vi "Read Header and Spreadsheet File.vi"(0 "DirIn":path=path "C:/ER2005/Data", 1 "NameIn":string="Test001.txt", 3 "Headers Only":bool, 4 "# Hdr Lines":i32=23 min=0, 5 "Error In":errorcluster, 6 "File Read Mode":enum16{"Never", "List", "Ask"}(ring)=enum."Ask", 8 "Delimiter (Tab)":string="\t", 10 "Format (%.4f)":string="%.4f", 11 "ErrMsgOff":bool, 13 "Transpose":bool) -> (12 "Table Out":string[][](array[string]), 14 "Filepath Out":path, 15 "File Text Out":string, 16 "Header Lines":string[](array[string]), 17 "Last 1D":sgl[](array[numeric]) format="%.2f", 18 "2D Data":sgl[][](array[numeric]) format="%.2f", 19 "Error Out":errorcluster)   [LabVIEW 2013]
panel:
  # "Err 1 - Invalid input parameter\nErr 4 - End-of-file\nErr 7 - Open error, file does not exist\nErr 43 - Cancel error"
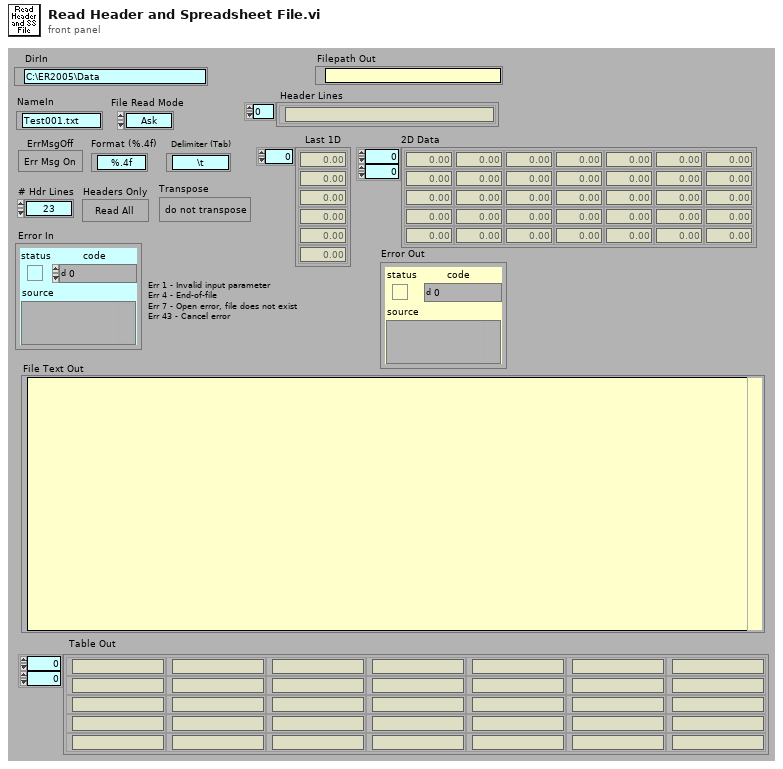
[diagram p1: front panel]
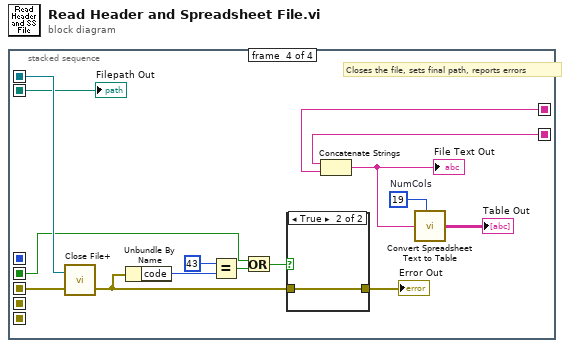
[diagram p0: block diagram]
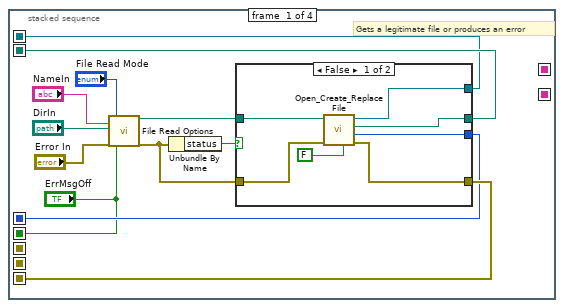
[diagram p2: hidden frame]
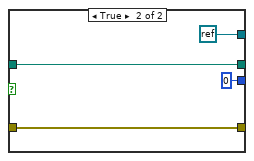
[diagram p3: hidden frame]
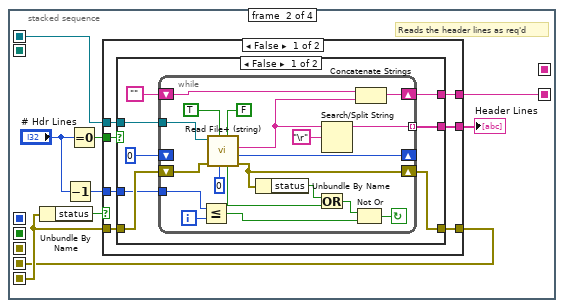
[diagram p4: hidden frame]
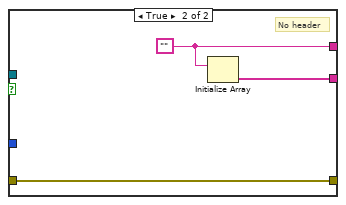
[diagram p5: hidden frame]
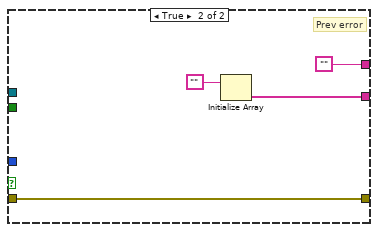
[diagram p6: hidden frame]
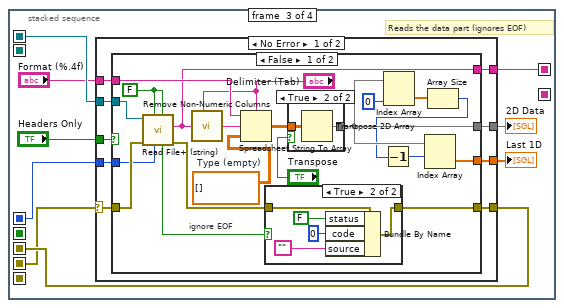
[diagram p7: hidden frame]
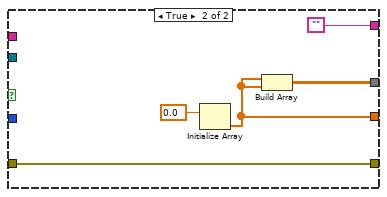
[diagram p10: hidden frame]
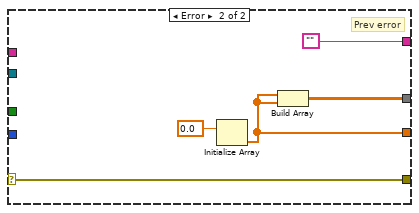
[diagram p11: hidden frame]
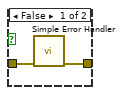
[diagram p12: hidden frame]
diagram:
  n1 = stacked-sequence {
    seq-local: [w5 _ _ _] -> [_ w31 _ _]
    seq-local: [w3 _ _ _] -> [_ w29 w81 w145]
    seq-local: [w4 _ _ _] -> [_ _ _ w144]
    seq-local: [_ w27 _ _] -> [_ _ w74 _]
    seq-local: [_ _ w82 _] -> [_ _ _ w143]
    seq-local: [w2 _ _ _] -> [_ _ w79 _]
    seq-local: ["ErrMsgOff" _ _ _] -> [_ _ _ w137]
    seq-local: [_ w24 _ _] -> [_ _ _ w135]
    seq-local: [_ _ w75 _] -> [_ _ _ w134]
    frame #0 {
      # "Gets a legitimate file or produces an error"
      n2 = call "File Read Options.vi"("NameIn"="NameIn", "DirIn"="DirIn", "ErrorIn (no error)"="Error In", "File Read Mode"="File Read Mode", "ErrMsgOff"="ErrMsgOff") -> ("PathOut"=w6:path, "ErrorOut"=w7:errorcluster)  [unwired: 7 in, 6 out]
      n3 = Unbundle By Name(w7) -> ("status"=w8:bool)
      n4 = case shown="False" w8 {
        tunnel: w6 -> [w19 w21]
        tunnel: [w16 w23] -> w5
        tunnel: w7 -> [w17 w23]
        tunnel: [w15 refnum<k0> refnum] -> w3
        tunnel: [w14 w21] -> w4
        tunnel: [w13 0 ("file size (bytes)")] -> w2
        frame False {
          n5 = call <vilib>:"Open_Create_Replace File.vi"("advisory dialog? (display:T)"=FALSE, "error in (no error)"=w17, "file path"=w19) -> ("error out"=w16:errorcluster, "file size (bytes)"=w13:i32, "new file path"=w14:path, "refnum"=w15:refnum<file>)  [unwired: 5 in]
        }
        frame True {
        }
      }
    }
    frame #1 {
      # "Reads the header lines as req'd"
      n6 = Unbundle By Name(w31) -> ("status"=w32:bool)
      n7 = Decrement(x="# Hdr Lines") -> (x-1=w25:i32)
      n8 = Equal To 0?(x="# Hdr Lines") -> (x = 0?=w30:bool)
      n9 = case shown="False" w32 {
        tunnel: w31 -> [w38 w71]
        tunnel: w25 -> [w37 _]
        tunnel: w30 -> [w39 _]
        tunnel: w29 -> [w36 _]
        tunnel: [w35 w72] -> w28
        tunnel: [w34 w71] -> w27
        tunnel: [w33 ""] -> w24
        frame False {
          n10 = case shown="False" w39 {
            tunnel: w38 -> [w46 w68]
            tunnel: w37 -> [w42 _]
            tunnel: w36 -> [w47 _]
            tunnel: [w44 w69] -> w35
            tunnel: [w43 w68] -> w34
            tunnel: [w40 w67] -> w33
            frame False {
              n11 = while {
                tunnel: w42 -> [w61]
                tunnel: [w51] -> w44 mode=indexing
                shift-left: 0 ("mark after read (bytes)") -> [_]
                shift-right: [w62] -> _
                shift-left: w46 -> [w63]
                shift-right: [w59] -> w43
                tunnel: w47 -> [w64]
                shift-right: [w50] -> w40
                shift-left: "" -> [w49]
                i -> [w60]
                stop <- w57 continue-if-true
                n12 = Less Or Equal?(x=w61, y=w60) -> (x <= y?=w58:bool)
                n13 = call <vilib>:"Read File+ (string).vi"("convert eol? (no:F)"=FALSE, "count"=0, "line mode (characters:F)"=TRUE, "error in (no error)"=w63, "refnum"=w64) -> ("error out"=w59:errorcluster, "mark after read (bytes)"=w62:i32, "string"=w48:string, "EOF?"=w56:bool)  [unwired: 2 in, 1 out]
                n14 = Unbundle By Name(w59) -> ("status"=w55:bool)
                n15 = Or(x=w55, y=w56) -> (x .or. y?=w54:bool)
                n16 = Search/Split String(string=w48, search string/char (-)="\r") -> (substring before match=w51:string)  [unwired: 1 in, 2 out]
                n17 = Not Or(1:w58, 2:w54) -> (0:w57:bool)
                n18 = Concatenate Strings(w49, w48) -> (w50:string)
              }
            }
            frame True {
              w67 = ""
              # "No header"
              n19 = Initialize Array(w67) -> (w69:string[])  [unwired: 1 in]
            }
          }
        }
        frame True {
          # "Prev error"
          n20 = Initialize Array("") -> (w72:string[])  [unwired: 1 in]
        }
      }
      "Header Lines" <- w28
    }
    frame #2 {
      # "Reads the data part (ignores EOF)"
      n21 = case shown="No Error" w74 {
        selector: w74 -> [w83 w126]
        tunnel: "Headers Only" -> [w91 _]
        tunnel: w81 -> [w90 _]
        tunnel: [w89 w126] -> w82
        tunnel: w79 -> [w88 _]
        tunnel: [w87 w129] -> w78
        tunnel: [w86 w128] -> w77
        tunnel: "Format (%.4f)" -> [w85 _]
        tunnel: [w84 ""] -> w75
        frame No Error {
          n22 = case shown="False" w91 {
            tunnel: w83 -> [w110 w125]
            tunnel: w90 -> [w111 _]
            tunnel: [w104 w125] -> w89
            tunnel: w88 -> [w109 _]
            tunnel: [w101 w122] -> w87
            tunnel: [w105 w123] -> w86
            tunnel: w85 -> [w95 _]
            tunnel: [w94 ""] -> w84
            frame False {
              w108 = sgl[][] []  # Type (empty)
              w96 = FALSE ("line mode (characters:F)")
              # "ignore EOF"
              n23 = call <vilib>:"Read File+ (string).vi"("convert eol? (no:F)"=w96, "count"=w109, "line mode (characters:F)"=w96, "error in (no error)"=w110, "refnum"=w111) -> ("error out"=w103:errorcluster, "string"=w94:string, "EOF?"=w102:bool)  [unwired: 2 in, 2 out]
              n24 = call "Remove Non-Numeric Columns.vi"("Separator (Tab)"="Delimiter (Tab)", "String In"=w94) -> ("String Out"=w93:string)  [unwired: 6 in, 1 out]
              n25 = Spreadsheet String To Array(delimiter (Tab)="Delimiter (Tab)", format string=w95, spreadsheet string=w93, array type (2D Dbl)=w108) -> (array=w107:sgl[][])
              n26 = case shown="True" w102 {
                tunnel: [w112 w116] -> w104
                tunnel: w103 -> [w112 w117]
                frame False {
                }
                frame True {
                  n27 = Bundle By Name(cluster=w117, "status"=FALSE ("Bundle Element"), "code"=0 ("Bundle Element"), "source"="") -> (w116:errorcluster)
                }
              }
              n28 = case shown="True" "Transpose" {
                tunnel: w107 -> [w118 w120]
                tunnel: [w118 w119] -> w101
                frame False {
                }
                frame True {
                  n29 = Transpose 2D Array(2D array=w120) -> (transposed array=w119:sgl[][])
                }
              }
              n30 = Index Array(array=w101, index (col)=0 ("disabled index (col)")) -> (element=w99:sgl[])  [unwired: 1 in]
              n31 = Array Size(array=w99) -> (size(s)=w98:i32)
              n32 = Decrement(x=w98) -> (x-1=w97:i32)
              n33 = Index Array(array=w101, index (row)=w97) -> (element=w105:sgl[])  [unwired: 1 in]
            }
            frame True {
              n34 = Initialize Array(sgl 0.0) -> (w123:sgl[])  [unwired: 1 in]
              n35 = Build Array(w123, w123) -> (w122:sgl[][])
            }
          }
        }
        frame Error {
          # "Prev error"
          n36 = Initialize Array(sgl 0.0) -> (w128:sgl[])  [unwired: 1 in]
          n37 = Build Array(w128, w128) -> (w129:sgl[][])
        }
      }
      "Last 1D" <- w77
      "2D Data" <- w78
    }
    frame #3 {
      w131 = 19  # NumCols
      # "Closes the file, sets final path, reports errors"
      n38 = call <vilib>:"Close File+.vi"("error in (no error)"=w143, "refnum"=w145) -> ("error out"=w141:errorcluster)  [unwired: 3 in, 2 out]
      n39 = Unbundle By Name(w141) -> ("code"=w140:i32)
      n40 = Equal?(x=43, y=w140) -> (x = y?=w138:bool)
      n41 = Or(x=w137, y=w138) -> (x .or. y?=w136:bool)
      n42 = case shown="True" w136 {
        tunnel: w141 -> [w147 w148]
        tunnel: [w146 w148] -> w142
        frame False {
          n43 = call <vilib>:"Simple Error Handler.vi"("error in (no error)"=w147) -> ("error out"=w146:errorcluster)  [unwired: 4 in, 4 out]
        }
        frame True {
        }
      }
      "Error Out" <- w142
      n44 = Concatenate Strings(w135, w134) -> (w133:string)
      "File Text Out" <- w133
      n45 = call "Convert Spreadsheet Text to Table.vi"("NumCols"=w131, "Text In"=w133) -> ("Table Out"=→"Table Out":string[][])  [unwired: 7 in]
      "Filepath Out" <- w144
    }
  }
